vi "FilterLittle_Direction.vi"(10 "Numeric":i32, 11 "Notifier in":refnum<notifier>) -> ()   [LabVIEW 2013]
doc: "When we know what 'direction' value indicates bad data, we can put that data into the test case and filter it out. It then won't be written up into the MidBrain, so only good data will be seen.\n\nEric Schneider, April 2014"
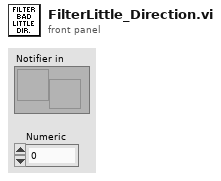
[diagram p1: front panel]
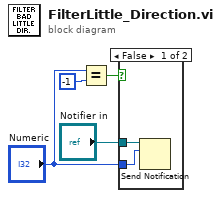
[diagram p0: block diagram]
diagram:
  n1 = Equal?(x="Numeric", y=-1) -> (x = y?=w2:bool)
  n2 = case shown="False" w2 {
    tunnel: "Notifier in" -> [w6 _]
    tunnel: "Numeric" -> [w5 _]
    frame False {
      n3 = Send Notification(notification=w5, notifier=w6) -> ()  [unwired: 1 in, 2 out]
    }
    frame True {
    }
  }
